vi "Set ni_measurementlink_measurement_v1_GetMetadataResponse.vi"(7 "Complete Call (T)":bool=TRUE, 8 "error in (no error)":errorcluster, 10 "package_templatemessage":T1, 11 "gRPCid":T9) -> (0 "error out":errorcluster)   [LabVIEW 2020, in "CancellableMeasurementProxy.lvlib"]
uses:
  CancellableMeasurementProxy.lvlib
  <vilib>/gRPC/LabVIEW gRPC Library/Shared/grpcId.ctl
  ni_measurementlink_measurement_v1_GetMetadataResponse.ctl
  ni_measurementlink_measurement_v1_MeasurementDetails.ctl
  ni_measurementlink_measurement_v1_MeasurementSignature.ctl
  ni_measurementlink_measurement_v1_ConfigurationParameter.ctl
  ni_measurementlink_measurement_v1_ConfigurationParameter_AnnotationsEntry.ctl
  google_protobuf_Any.ctl
  ni_measurementlink_measurement_v1_Output.ctl
  ni_measurementlink_measurement_v1_UserInterfaceDetails.ctl
  dcc74a39-081a-4bdd-860b-8ed792803c96.vi
  <vilib>/gRPC/LabVIEW gRPC Library/Shared/TranslateGrpcError.vi
  <vilib>/gRPC/LabVIEW gRPC Library/Server API/Server/Get Server DLL Path.vi
  <vilib>/Utility/error.llb/Error Cluster From Error Code.vi
  <vilib>/gRPC/LabVIEW gRPC Library/grpc-lvsupport-release.lvlib
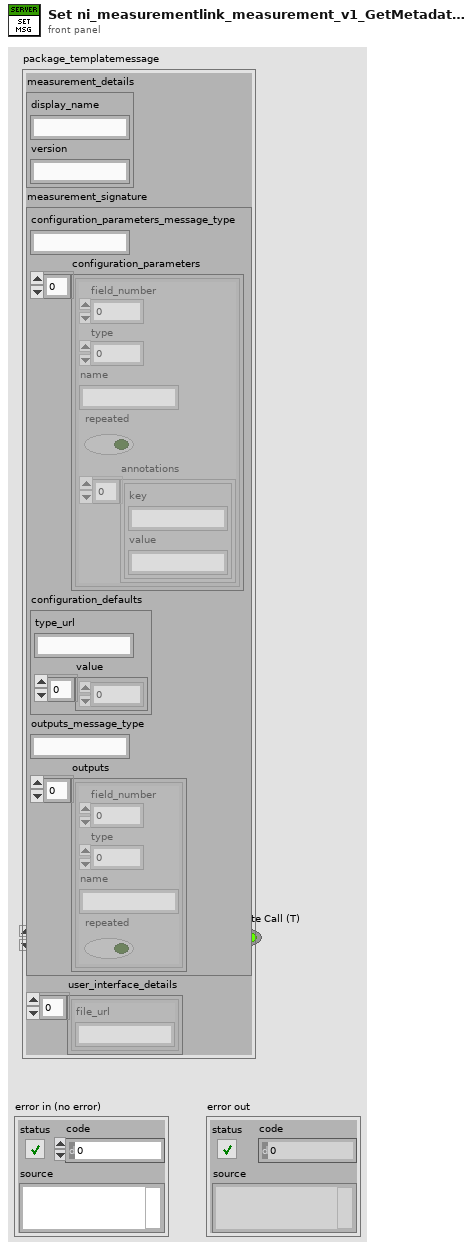
[diagram p1: front panel]
types:
  T1 = typedef "CancellableMeasurementProxy.lvlib/ni_measurementlink_measurement_v1_GetMetadataResponse.ctl" = cluster{"measurement_details":T2, "measurement_signature":T3, "user_interface_details":T8[]}
  T2 = typedef "CancellableMeasurementProxy.lvlib/ni_measurementlink_measurement_v1_MeasurementDetails.ctl" = cluster{"display_name":string, "version":string}
  T3 = typedef "CancellableMeasurementProxy.lvlib/ni_measurementlink_measurement_v1_MeasurementSignature.ctl" = cluster{"configuration_parameters_message_type":string, "configuration_parameters":T4[], "configuration_defaults":T6, "outputs_message_type":string, "outputs":T7[]}
  T4 = typedef "CancellableMeasurementProxy.lvlib/ni_measurementlink_measurement_v1_ConfigurationParameter.ctl" = cluster{"field_number":i32, "type":i32, "name":string, "repeated":bool, "annotations":T5[]}
  T5 = typedef "CancellableMeasurementProxy.lvlib/ni_measurementlink_measurement_v1_ConfigurationParameter_AnnotationsEntry.ctl" = cluster{"key":string, "value":string}
  T6 = typedef "CancellableMeasurementProxy.lvlib/google_protobuf_Any.ctl" = cluster{"type_url":string, "value":u8[]}
  T7 = typedef "CancellableMeasurementProxy.lvlib/ni_measurementlink_measurement_v1_Output.ctl" = cluster{"field_number":i32, "type":i32, "name":string, "repeated":bool}
  T8 = typedef "CancellableMeasurementProxy.lvlib/ni_measurementlink_measurement_v1_UserInterfaceDetails.ctl" = cluster{"file_url":string}
  T9 = typedef "grpc-lvsupport-release.lvlib/grpcId.ctl" = u64
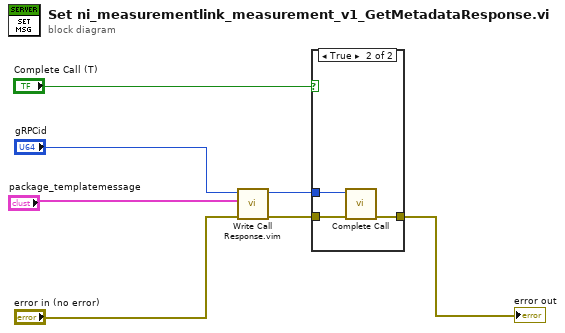
[diagram p0: block diagram]
diagram:
  n1 = call "Write Call Response.vim"("error in"="error in (no error)", "Response Data"="package_templatemessage", "gRPCid in"="gRPCid") -> ("error out"=w4:errorcluster, "gRPCid out"=w5:T9)  [unwired: 7 in]
  n2 = case shown="True" "Complete Call (T)" {
    tunnel: [w8 w11] -> w7
    tunnel: w5 -> [_ w10]
    tunnel: w4 -> [w8 w9]
    frame False {
    }
    frame True {
      n3 = call <vilib>:"Complete Call.vi"("gRPCid"=w10, "error in"=w9) -> ("error out"=w11:errorcluster)  [unwired: 8 in]
    }
  }
  "error out" <- w7
